vi "EacExperiment.vi"(0 "object in":refnum<class "SaveData.lvclass">, 1 "Path":path, 2 "Temperature (C)":dbl, 3 "Oscilloscope Results":T2 {"Probe Current" format="%.2p"; "Phase Angle" format="%.2p"; "Main Freq" format="%.2p"; "Main Volt" format="%.2p"; "Prefocus Freq" format="%.2p"; "Prefocus Volt" format="%.2p"}, 4 "Experiment Settings":T1={"Frequencies (MHz)"=[], "Camera Settings"={"Minimum Time between\n frames(s)"=10.0, "Number of Frames"=0}, "Flowrates (ul/min)"=[], "Voltages (V)"=[]} {"Camera Settings"."Minimum Time between\n frames(s)" min=0.005}, 5 "error in (no error)":errorcluster) -> (14 "object out":refnum<class "SaveData.lvclass">, 19 "error out":errorcluster)   [LabVIEW 2023, in "SaveData.lvclass"]
uses:
  SaveData.lvclass
  <vilib>/express/express shared/transition.llb/Dynamic To Waveform Array.vi
  <vilib>/express/express signal manip/GetorSetDDTAttributes/Set DDT Attributes/SetT0.vi
  <vilib>/express/express shared/transition.llb/Waveform Array To Dynamic.vi
  <vilib>/express/express signal manip/GetorSetDDTAttributes/Set DDT Attributes/Set DDT Properties.xnode
  SaveData.lvclass/SaveData.ctl
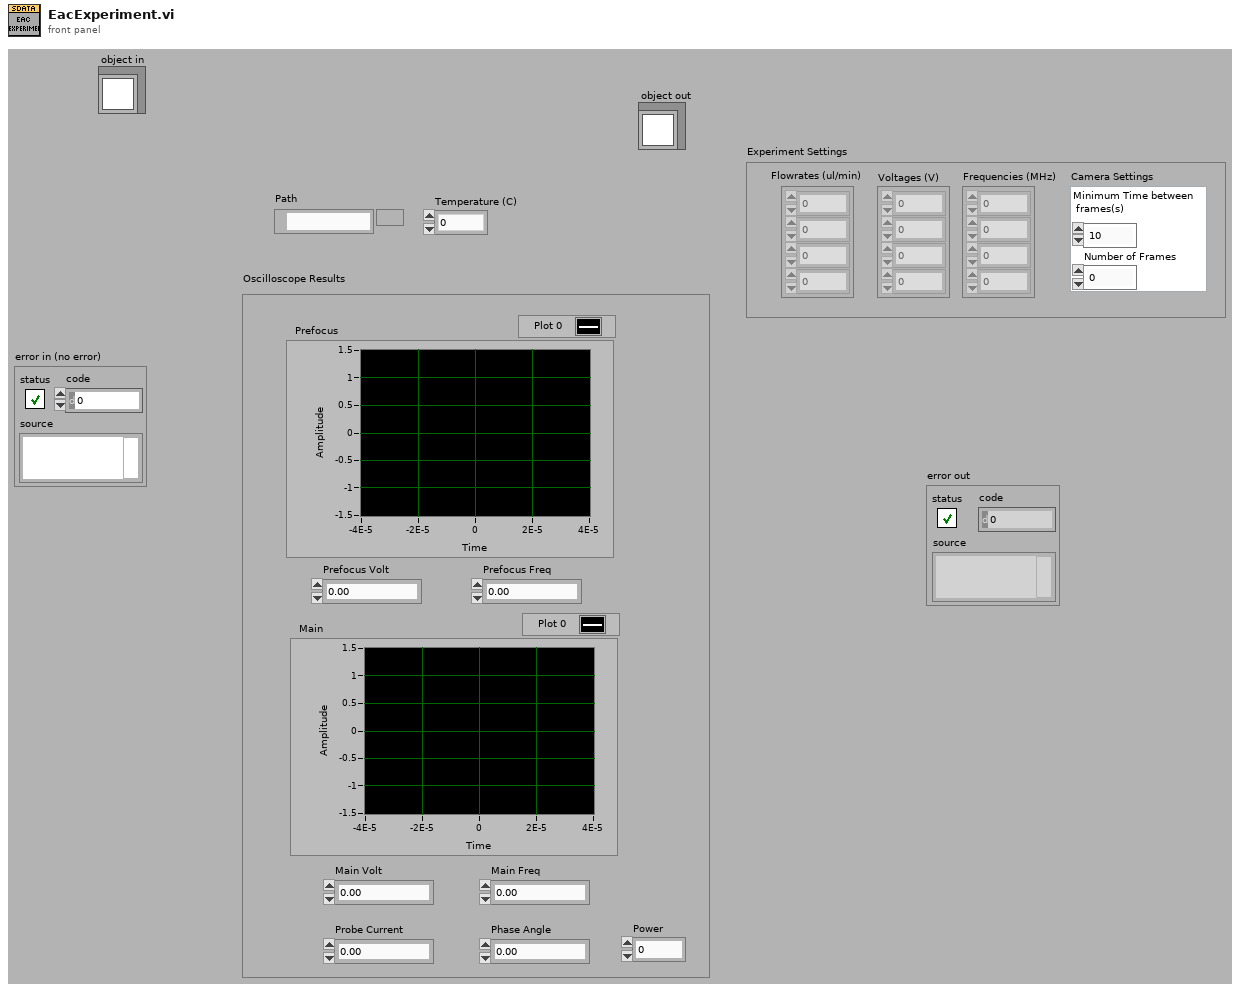
[diagram p1: front panel]
types:
  T1 = cluster{"Frequencies (MHz)":dbl[], "Camera Settings":cluster{"Minimum Time between\n frames(s)":dbl, "Number of Frames":i32}, "Flowrates (ul/min)":dbl[], "Voltages (V)":dbl[]}
  T2 = cluster{"Prefocus":cluster{"Initial X":dbl, "X Increment":dbl, "Waveform Array":dbl[]}, "Prefocus Volt":dbl, "Prefocus Freq":dbl, "Main":cluster{"Initial X":dbl, "X Increment":dbl, "Waveform Array":dbl[]}, "Main Volt":dbl, "Main Freq":dbl, "Phase Angle":dbl, "Probe Current":dbl, "Power":dbl}
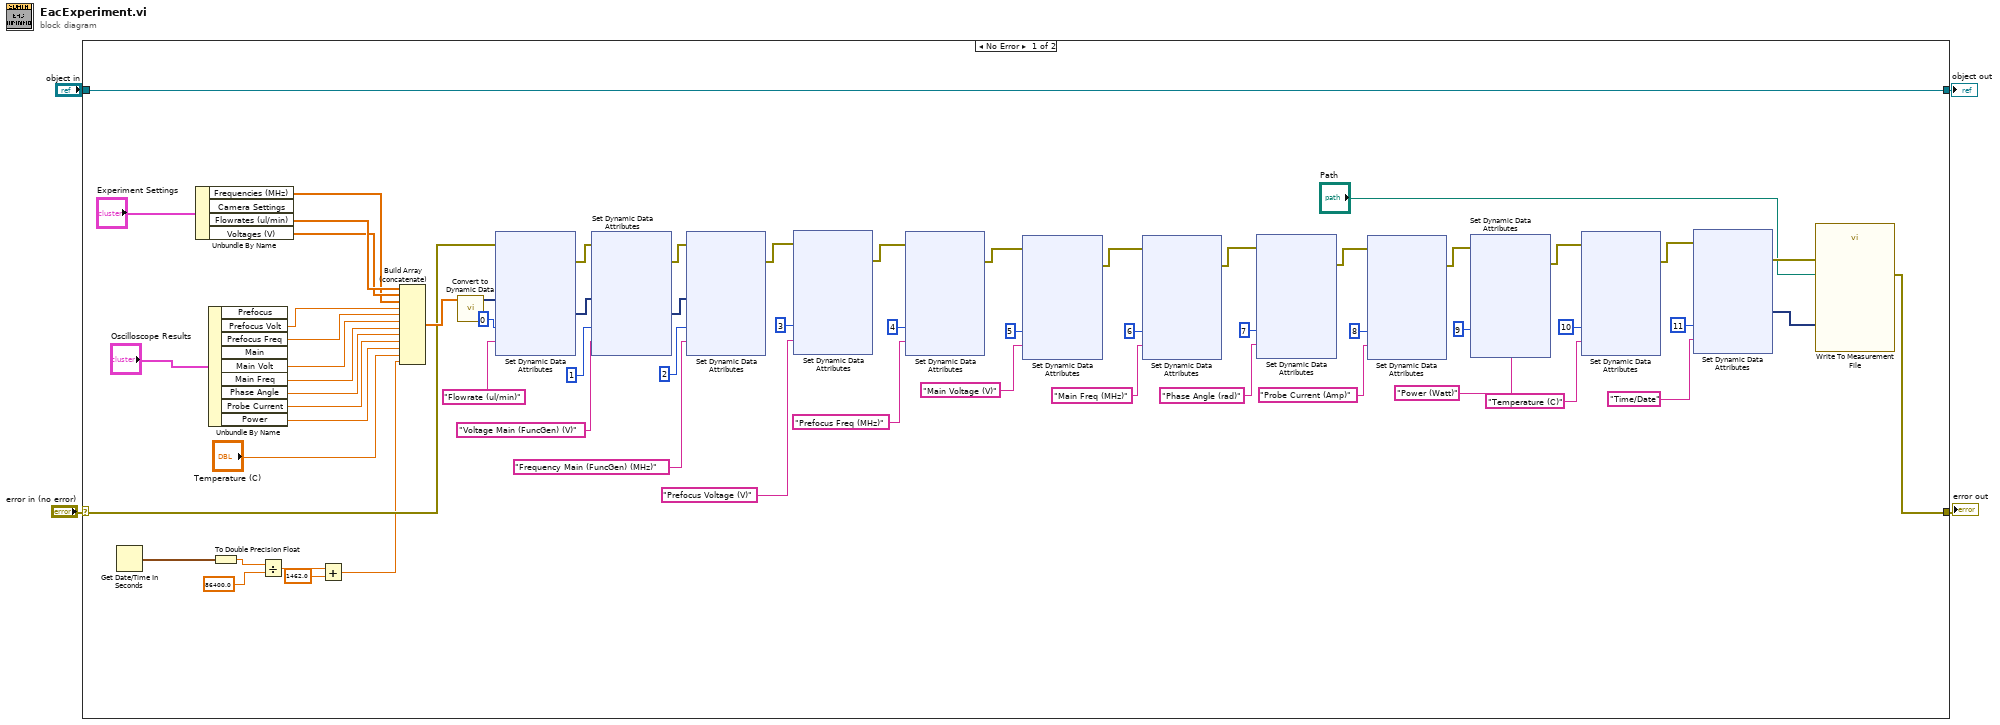
[diagram p0: block diagram]
diagram:
  n1 = case shown="No Error" "error in (no error)" {
    selector: "error in (no error)" -> [w32 w226]
    tunnel: [w31 w226] -> w3
    tunnel: [w68 w225] -> w1
    tunnel: "object in" -> [w68 w225]
    frame No Error {
      n2 = Get Date/Time In Seconds() -> (seconds since 1Jan1904=w46:timestamp)
      n3 = Unbundle By Name("Experiment Settings") -> ("Frequencies (MHz)"=w49:dbl[], "Flowrates (ul/min)"=w51:dbl[], "Voltages (V)"=w50:dbl[])  [unwired: 1 out]
      n4 = Unbundle By Name("Oscilloscope Results") -> ("Prefocus Volt"=w18:dbl, "Prefocus Freq"=w17:dbl, "Main Volt"=w16:dbl, "Main Freq"=w15:dbl, "Phase Angle"=w48:dbl, "Probe Current"=w47:dbl, "Power"=w10:dbl)  [unwired: 2 out]
      n5 = To Double Precision Float(number=w46) -> (double precision float=w45:dbl)
      n6 = Divide(x=w45, y=86400.0) -> (x/y=w43:dbl)
      n7 = Add(x=w43, y=1462.0) -> (x+y=w8:dbl)
      n8 = Build Array (concatenate)(w51, w50, w49, w18, w17, w16, w15, w48, w47, w10, "Temperature (C)", w8) -> (w67:dbl[])
      n9 = call "Convert to Dynamic Data"("Array"=w67) -> ("Dynamic Data Type"=w66:dynamicdata)  [unwired: 3 in]
      n10 = xnode "Set Dynamic Data Attributes"("Signals In"=w66, "Signal Index"=0, "Signal Name"="Flowrate (ul/min)", "error in"=w32) -> ("Signals Out"=w61:dynamicdata, "error out"=w54:errorcluster)
      n11 = xnode "Set Dynamic Data Attributes"("Signals In"=w61, "Signal Index"=1, "Signal Name"="Voltage Main (FuncGen) (V)", "error in"=w54) -> ("Signals Out"=w58:dynamicdata, "error out"=w55:errorcluster)
      n12 = xnode "Set Dynamic Data Attributes"("Signals In"=w58, "Signal Index"=2, "Signal Name"="Frequency Main (FuncGen) (MHz)", "error in"=w55) -> ("error out"=w41:errorcluster)  [unwired: 1 out]
      n13 = xnode "Set Dynamic Data Attributes"("Signal Index"=3, "Signal Name"="Prefocus Voltage (V)", "error in"=w41) -> ("error out"=w40:errorcluster)  [unwired: 1 in, 1 out]
      n14 = xnode "Set Dynamic Data Attributes"("Signal Index"=4, "Signal Name"="Prefocus Freq (MHz)", "error in"=w40) -> ("error out"=w39:errorcluster)  [unwired: 1 in, 1 out]
      n15 = xnode "Set Dynamic Data Attributes"("Signal Index"=5, "Signal Name"="Main Voltage (V)", "error in"=w39) -> ("error out"=w38:errorcluster)  [unwired: 1 in, 1 out]
      n16 = xnode "Set Dynamic Data Attributes"("Signal Index"=6, "Signal Name"="Main Freq (MHz)", "error in"=w38) -> ("error out"=w37:errorcluster)  [unwired: 1 in, 1 out]
      n17 = xnode "Set Dynamic Data Attributes"("Signal Index"=7, "Signal Name"="Phase Angle (rad)", "error in"=w37) -> ("error out"=w36:errorcluster)  [unwired: 1 in, 1 out]
      n18 = xnode "Set Dynamic Data Attributes"("Signal Index"=8, "Signal Name"="Probe Current (Amp)", "error in"=w36) -> ("error out"=w35:errorcluster)  [unwired: 1 in, 1 out]
      n19 = xnode "Set Dynamic Data Attributes"("Signal Index"=9, "Signal Name"="Power (Watt)", "error in"=w35) -> ("error out"=w34:errorcluster)  [unwired: 1 in, 1 out]
      n20 = xnode "Set Dynamic Data Attributes"("Signal Index"=10, "Signal Name"="Temperature (C)", "error in"=w34) -> ("error out"=w33:errorcluster)  [unwired: 1 in, 1 out]
      n21 = xnode "Set Dynamic Data Attributes"("Signal Index"=11, "Signal Name"="Time/Date", "error in"=w33) -> ("Signals Out"=w57:dynamicdata, "error out"=w56:errorcluster)  [unwired: 1 in]
      n22 = call "Write To Measurement File"("Signals"=w57, "error in (no error)"=w56, "Filename"="Path") -> ("error out"=w31:errorcluster)  [unwired: 14 in, 2 out]
    }
    frame Error {
    }
  }
  "error out" <- w3
  "object out" <- w1
